vi "6221+2182.vi"() -> ()   [LabVIEW 2019]
uses:
  <vilib>/Utility/file.llb/Write Delimited Spreadsheet (DBL).vi
  lib/Keithley 2182/Keithley 2182.lvlib
  lib/Keithley 622x/Keithley 622x.lvlib
panel:
  in  "delay (ms)":u32=500
  in  "2182":refnum<visa-resource-name>="GPIB1::7::INSTR"
  in  "6221":refnum<visa-resource-name>="GPIB0::24::INSTR"
  in  "Instrument Type":i32(ring)=3 items=["PPMS", "VersaLab", "DynaCool", "SVSM"]
  out "Measurement Metadata":T1
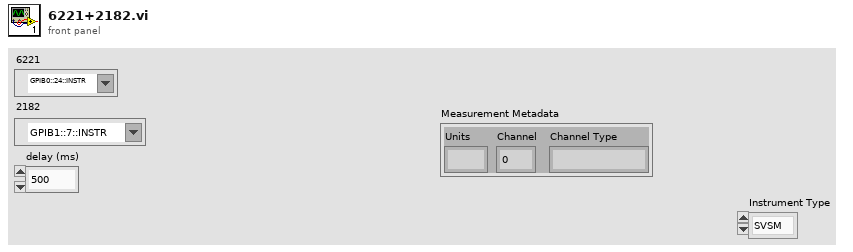
[diagram p1: front panel]
types:
  T1 = cluster{"Units":string, "Channel":i32, "Channel Type":string}
  T2 = enum16{"open", "replace", "create", "open or create", "replace or create", "replace or create with confirmation"}
  T3 = typedef "Keithley 622x.lvlib/KE622x -- Current Level.ctl" = dbl
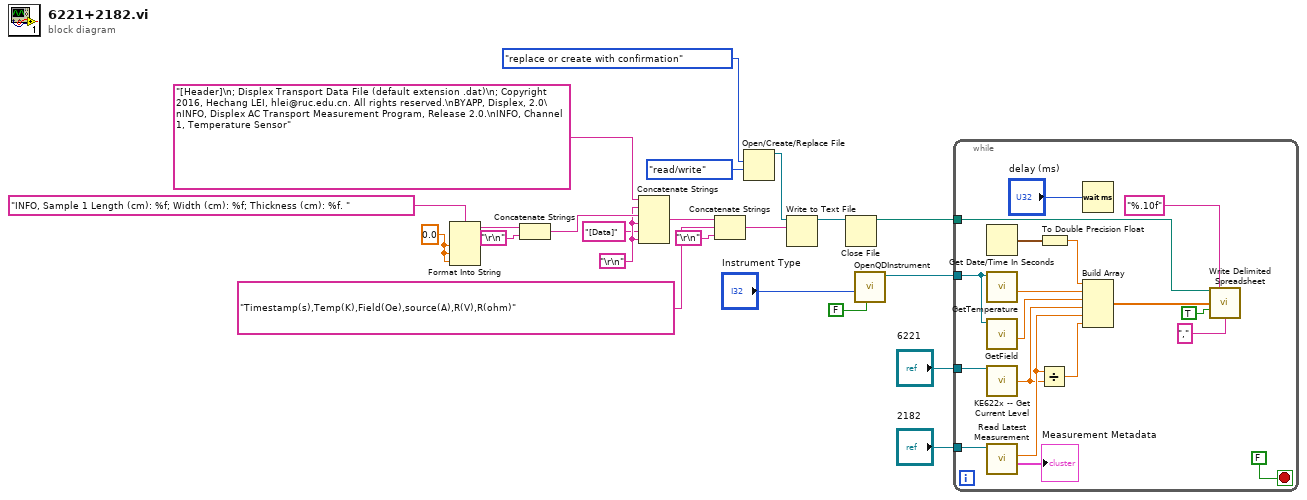
[diagram p0: block diagram]
diagram:
  w18 = 0.0 ("输入 1")
  w15 = "\r\n"
  n1 = Format Into String(format string="INFO, Sample 1 Length (cm): %f; Width (cm): %f; Thickness (cm): %f. " ("string"), w18, w18, w18) -> (resulting string=w20:string)  [unwired: 2 in, 1 out]
  n2 = Concatenate Strings(w20, "\r\n") -> (w22:string)
  n3 = Concatenate Strings("[Header]\n; Displex Transport Data File (default extension .dat)\n; Copyright 2016, Hechang LEI, hlei@ruc.edu.cn. All rights reserved.\nBYAPP, Displex, 2.0\nINFO, Displex AC Transport Measurement Program, Release 2.0.\nINFO, Channel 1, Temperature Sensor" ("string"), w15, w22, w15, "[Data]" ("string"), w15) -> (w21:string)
  n4 = Concatenate Strings(w21, "Timestamp(s),Temp(K),Field(Oe),source(A),R(V),R(ohm)" ("字符串"), "\r\n") -> (w12:string)
  n5 = Open/Create/Replace File(operation (0:open)=T2."replace or create with confirmation" ("操作(0:open)"), access (0:read/write)=enum16{"read/write", "read-only", "write-only"}."read/write" ("权限(0:read/write)")) -> (refnum out=w11:refnum<file>)  [unwired: 4 in, 2 out]
  n6 = Write to Text File(file (use dialog)=w11, text=w12) -> (refnum out=w8:refnum<file>)  [unwired: 2 in, 2 out]
  n7 = Close File(refnum=w8) -> (path=w6:path)  [unwired: 1 in, 1 out]
  n8 = call "OpenQDInstrument.vi"("Remote"=FALSE, "Instrument Type"="Instrument Type") -> ("Instrument Ref"=w1:refnum<k24>)  [unwired: 6 in, 1 out]
  n9 = while {
    tunnel: w6 -> [w32]
    tunnel: "6221" -> [w31]
    tunnel: "2182" -> [w26]
    tunnel: w1 -> [w23]
    stop <- FALSE stop-if-true
    n10 = Get Date/Time In Seconds() -> (seconds since 1Jan1904=w36:timestamp)
    n11 = call "GetTemperature.vi"("Instrument Ref In"=w23) -> ("Temperature"=w40:dbl)  [unwired: 4 in, 4 out]
    n12 = call "GetField.vi"("Instrument Ref In"=w23) -> ("Field"=w39:dbl)  [unwired: 4 in, 4 out]
    n13 = call "KE622x -- Get Current Level.vi"("Resource In"=w31) -> ("Current Level (A)"=w29:T3)  [unwired: 12 in, 2 out]
    n14 = call "Read Latest Measurement.vi"("VISA resource name"=w26) -> ("Measurement Metadata"=→"Measurement Metadata":T1, "Measurement"=w30:dbl)  [unwired: 7 in, 2 out]
    n15 = Divide(x=w30, y=w29) -> (x/y=w28:T3)
    n16 = To Double Precision Float(number=w36) -> (double precision float=w35:dbl)
    n17 = Wait (ms)(milliseconds to wait="delay (ms)") -> ()  [unwired: 1 out]
    n18 = Build Array(w35, w40, w39, w29, w30, w28) -> (w34:T3[])
    n19 = call-poly <vilib>:"Write Delimited Spreadsheet.vi"("file path (dialog if empty)"=w32, "format (%.3f)"="%.10f", "1D data"=w34, "append to file? (new file:F)"=TRUE, "delimiter (\\t)"="," ("delimiter (\\t)")) -> ()  [unwired: 9 in, 2 out]
  }
